vi "Unregister From Hotel.vi"(9 "hotel":string, 10 "guest":string, 11 "map in":map{string, set{string}}(c390)) -> (1 "removed last registration?":bool, 2 "guest not registered for this hotel?":bool, 3 "map out":map{string, set{string}}(c390))   [LabVIEW 2023]
doc: "This VI unregisters a guest from the given hotel."
uses:
  a640a025-6799-4771-87b0-58839cf4e77c.vi
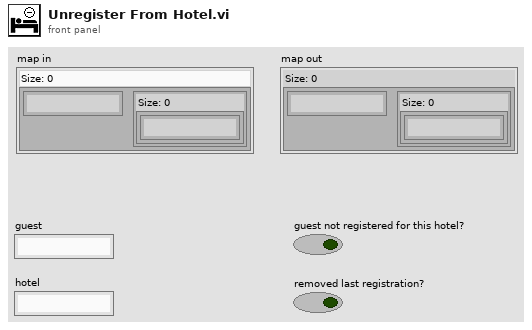
[diagram p1: front panel]
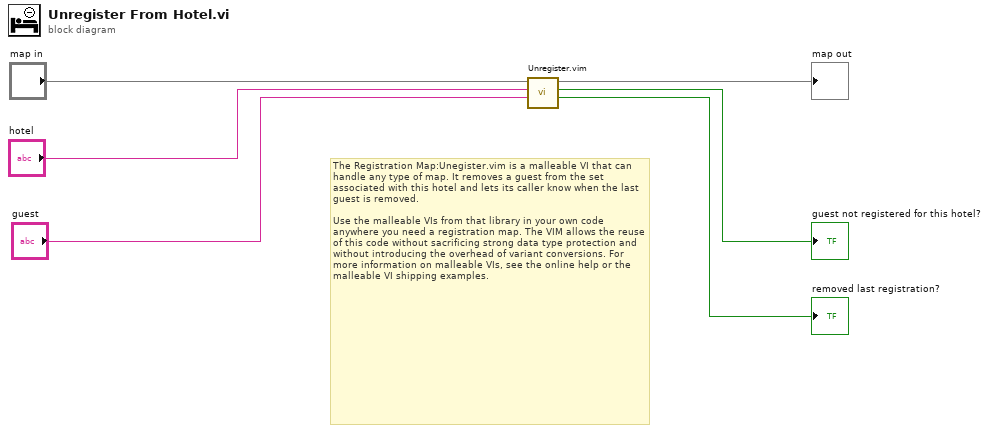
[diagram p0: block diagram]
diagram:
  # "The Registration Map:Unegister.vim is a malleable VI that can handle any type of map. It removes a guest from the set associated with this hotel and lets its caller know when the last guest is removed. \n\nUse the malleable VIs from that library in your own code anywhere you need a registration map. The VIM allows the reuse of this code without sacrificing strong data type protection and without introducing the overhead of variant conversions. For more information on malleable VIs, see the online help or the malleable VI shipping examples."
  n1 = call "Unregister.vim"("set element"="guest", "key"="hotel", "map in"="map in") -> ("removed last registration for this key?"=→"removed last registration?":bool, "element not registered for this key?"=→"guest not registered for this hotel?":bool, "map out"=→"map out":map{string, set{string}})  [unwired: 6 in]
